vi "Queue Driver.vi"(0 "Queue Name":string, 5 "States[]":string[](array[string]), 11 "Error In":errorcluster, 13 "Queue Operation":T1) -> (4 "Dequeue Element":string, 15 "Error Out":errorcluster)   [LabVIEW 2023]
doc: "The VI performs the queue operations. The operations include create, enqueue, dequeue, flush and closes the queue."
uses:
  Typedef/Queue Operation.ctl
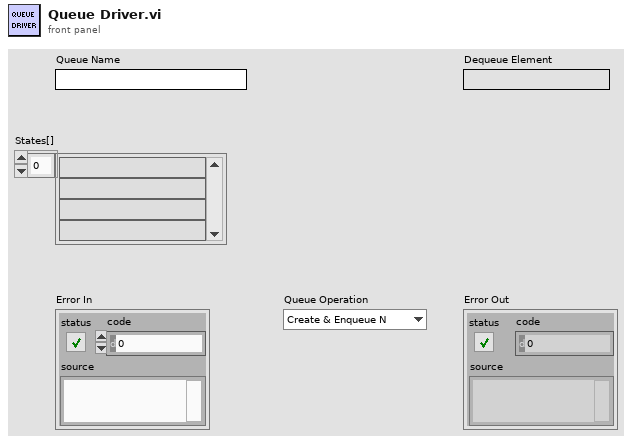
[diagram p1: front panel]
types:
  T1 = typedef "Queue Operation.ctl" = enum16{"Create & Enqueue N", "Enqueue N", "Dequeue", "Enstack N", "Flush", "Release"}
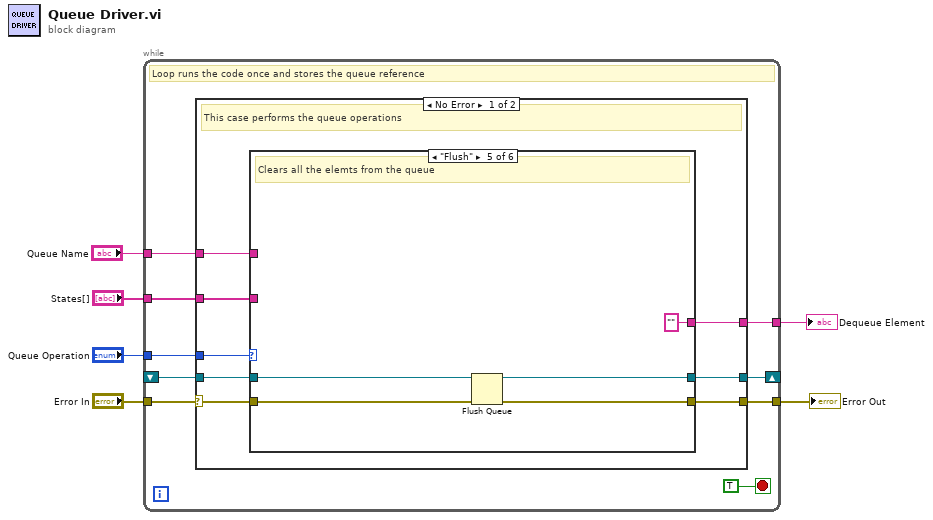
[diagram p0: block diagram]
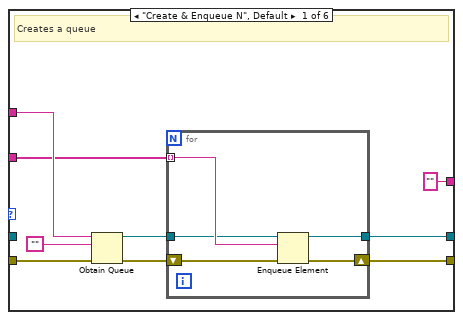
[diagram p2: hidden frame]
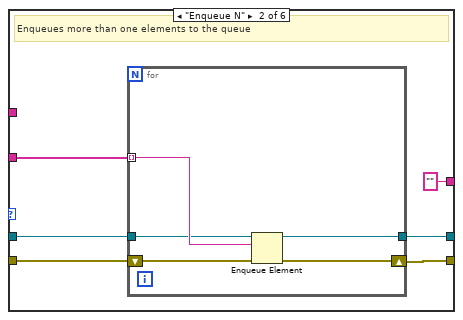
[diagram p3: hidden frame]
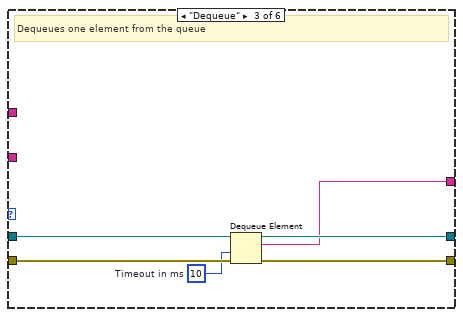
[diagram p4: hidden frame]
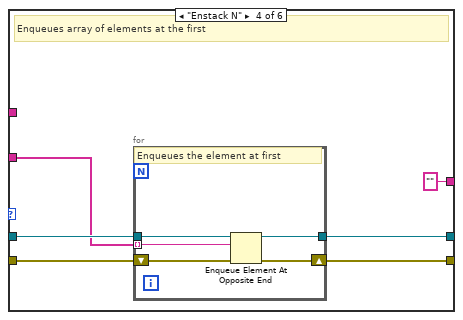
[diagram p5: hidden frame]
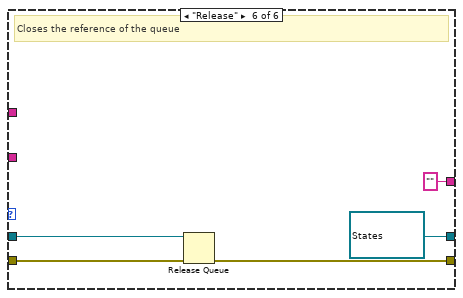
[diagram p6: hidden frame]
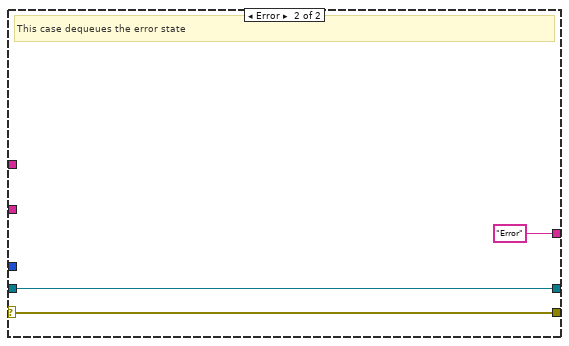
[diagram p7: hidden frame]
diagram:
  n1 = while {
    tunnel: "Error In" -> [w15]
    tunnel: "Queue Operation" -> [w14]
    tunnel: "Queue Name" -> [w13]
    tunnel: "States[]" -> [w12]
    shift-right: [w11] -> _
    shift-left: _ -> [w10]
    tunnel: [w9] -> w2
    tunnel: [w7] -> w1
    stop <- TRUE stop-if-true
    # "Loop runs the code once and stores the queue reference"
    n2 = case shown="No Error" w15 {
      selector: w15 -> [w23 w77]
      tunnel: w14 -> [w22 _]
      tunnel: w13 -> [w21 _]
      tunnel: w12 -> [w20 _]
      tunnel: [w19 w78] -> w11
      tunnel: w10 -> [w18 w78]
      tunnel: [w17 w77] -> w9
      tunnel: [w16 "Error" ("Queue Name")] -> w7
      frame No Error {
        # "This case performs the queue operations"
        n3 = case shown="\"Flush\"" w22 {
          tunnel: [w26 w42 w53 w59 w69 w74] -> w17
          tunnel: w23 -> [w32 w43 w54 w60 w70 w75]
          tunnel: w21 -> [w31 _ _ _ _ _]
          tunnel: w20 -> [w29 w41 _ w55 _ _]
          tunnel: [w27 w39 w52 w57 w67 refnum<queue> refnum ("queue out")] -> w19
          tunnel: w18 -> [_ w40 w51 w58 w68 w73]
          tunnel: ["" ("States") "" ("States") w49 "" ("States") "" ("States") "" ("States")] -> w16
          frame "Create & Enqueue N", Default {
            # "Creates a queue"
            n4 = Obtain Queue(name (unnamed)=w31, element data type="", error in (no error)=w32) -> (queue out=w28:refnum<queue>, error out=w25:errorcluster)  [unwired: 2 in, 1 out]
            n5 = for {
              shift-right: [w36] -> w26
              shift-left: w25 -> [w37]
              tunnel: w29 -> [w35] mode=indexing
              tunnel: w28 -> [w34]
              tunnel: [w33] -> w27
              n6 = Enqueue Element(queue=w34, element=w35, error in (no error)=w37) -> (queue out=w33:refnum<queue>, error out=w36:errorcluster)  [unwired: 1 in, 1 out]
            }
          }
          frame "Enqueue N" {
            # "Enqueues more than one elements to the queue"
            n7 = for {
              shift-right: [w47] -> w42
              shift-left: w43 -> [w48]
              tunnel: w41 -> [w46] mode=indexing
              tunnel: w40 -> [w45]
              tunnel: [w44] -> w39
              n8 = Enqueue Element(queue=w45, element=w46, error in (no error)=w48) -> (queue out=w44:refnum<queue>, error out=w47:errorcluster)  [unwired: 1 in, 1 out]
            }
          }
          frame "Dequeue" {
            w50 = 10  # Timeout in ms
            # "Dequeues one element from the queue"
            n9 = Dequeue Element(queue=w51, timeout in ms (-1)=w50, error in (no error)=w54) -> (queue out=w52:refnum<queue>, element=w49:string, error out=w53:errorcluster)  [unwired: 1 out]
          }
          frame "Enstack N" {
            # "Enqueues array of elements at the first"
            n10 = for {
              tunnel: w58 -> [w63]
              tunnel: [w62] -> w57
              tunnel: w55 -> [w61] mode=indexing
              shift-right: [w64] -> w59
              shift-left: w60 -> [w65]
              # "Enqueues the element at first"
              n11 = Enqueue Element At Opposite End(queue=w63, element=w61, error in (no error)=w65) -> (queue out=w62:refnum<queue>, error out=w64:errorcluster)  [unwired: 1 in, 1 out]
            }
          }
          frame "Flush" {
            # "Clears all the elemts from the queue"
            n12 = Flush Queue(queue=w68, error in (no error)=w70) -> (queue out=w67:refnum<queue>, error out=w69:errorcluster)  [unwired: 1 out]
          }
          frame "Release" {
            # "Closes the reference of the queue"
            n13 = Release Queue(queue=w73, error in (no error)=w75) -> (error out=w74:errorcluster)  [unwired: 1 in, 2 out]
          }
        }
      }
      frame Error {
        # "This case dequeues the error state"
      }
    }
  }
  "Error Out" <- w2
  "Dequeue Element" <- w1
